vi "Not A Timer.vi"(1 "timer":T1) -> (0 "not a timer":bool)   [LabVIEW 2011]
doc: "Returns TRUE if timer is not a valid timer refnum.\n\n© Copyright 1999\nCal-Bay Systems, Inc.\nwritten by James Kring"
uses:
  Timer Refnum.ctl
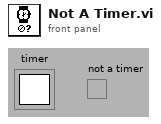
[diagram p1: front panel]
types:
  T1 = typedef "Timer Refnum.ctl" = refnum<k1>
  T2 = enum16{"open ref", "lookup ref", "close ref", "test ref", "start", "stop", "wait", "reset", "increment # waiting", "decrement #waiting"}
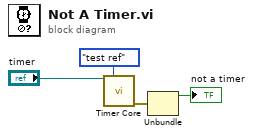
[diagram p0: block diagram]
diagram:
  n1 = call "Timer Core.vi"("timer"="timer", "function"=T2."test ref") -> ("error out"=w3:errorcluster)  [unwired: 7 in, 6 out]
  n2 = Unbundle(w3) -> ("status"=→"not a timer":bool)  [unwired: 2 out]
